vi "StartClone.vi"(7 "ShowPanel? (f)":bool, 8 "error in (no error)":errorcluster, 10 "ModuleName":string="unnamed", 11 "VI Refnum":refnum<vi>) -> (0 "error out":errorcluster, 1 "clBroadcastEvents":T1, 3 "ModuleAdmin":refnum<class "ModuleAdmin.lvclass">)   [LabVIEW 2018, in "SensorModule.lvlib"]
uses:
  SensorModule.lvlib
  SensorShared/clBroadcastEvents.ctl
  SensorShared/clEventType.ctl
  <userlib>/NIST/ModuleAdminLib/ModuleAdmin/ModuleAdmin.lvclass
  C:/Program Files (x86)/National Instruments/LabVIEW 2018/user.lib/NIST/ModuleAdminLib/ModuleAdminBase/ModuleAdminBase.lvclass
  <userlib>/NIST/ModuleAdminLib/ModuleAdmin/ModuleAdmin.lvclass/ModuleAdmin.ctl
  <userlib>/NIST/ModuleAdminLib/ModuleAdmin/Accessors/Write CloneRegRef.vi
  <userlib>/NIST/ModuleAdminLib/ModuleAdmin/Accessors/Write ShowPanel_.vi
  <vilib>/Utility/error.llb/Error Cluster From Error Code.vi
  <vilib>/ErrorRing/Error Ring.xnode
  SensorShared/SensorShared.lvlib
  <userlib>/NIST/ModuleAdminLib/ModuleAdminBase/ModuleAdminBase.lvclass
  <userlib>/NIST/ModuleAdminLib/CloneRegistration/CloneRegistration.lvclass
panel:
  # "If you want to add other Broadcast Events, open this typedef, copy an existing event and rename it to your event name.\n\nNext create an \"arg\" typedef for the  data and put it into PublicAPI/Arguments/Broadcasts\n\nAfter that, you will need to create a new roadcast vi in Protected/Broadcast.  Look at DidInit.vi or the reportError.vi as examples."
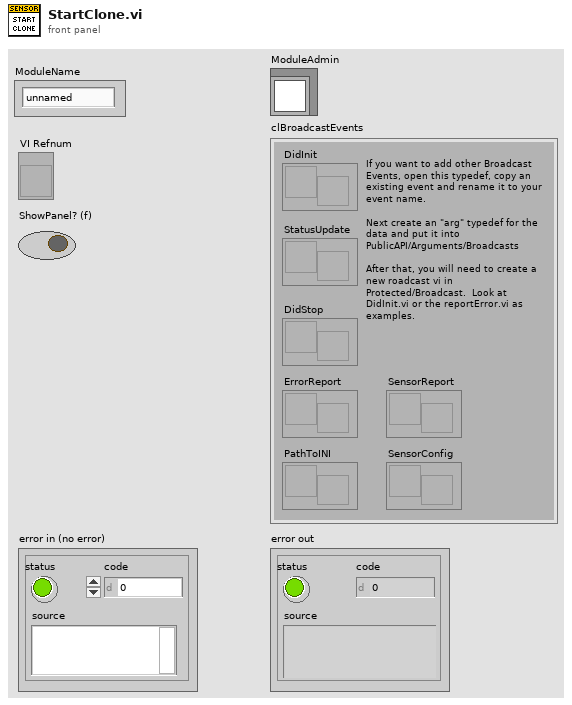
[diagram p1: front panel]
types:
  T1 = typedef "SensorShared.lvlib/clBroadcastEvents.ctl" = cluster{"DidInit":refnum<user-event>, "StatusUpdate":refnum<user-event>, "ErrorReport":refnum<user-event>, "DidStop":refnum<user-event>, "PathToINI":refnum<user-event>, "SensorReport":refnum<user-event>, "SensorConfig":refnum<user-event>}
  T2 = enum32{"Bad", "Idle", "Run top level", "Running"}
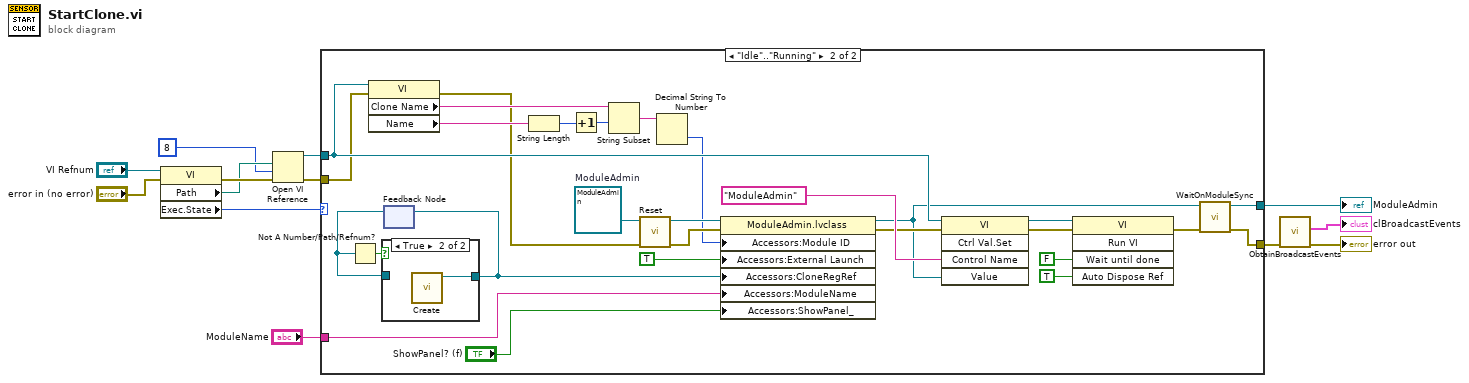
[diagram p0: block diagram]
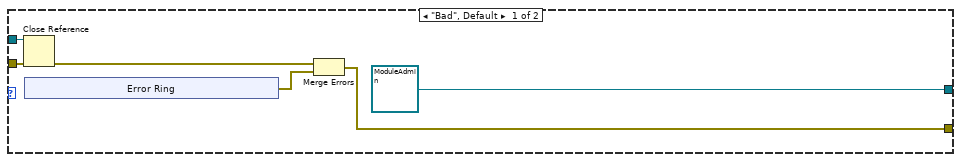
[diagram p2: hidden frame]
diagram:
  n1 = property class="VI"(reference="VI Refnum", error in="error in (no error)") -> (error out=w11:errorcluster, "Path"=w10:path, "Exec.State"=w12:T2)  [unwired: 1 out]
  n2 = Open VI Reference(vi path=w10, options=8, error in (no error)=w11) -> (vi reference=w8:refnum<vi>, error out=w9:errorcluster)  [unwired: 3 in]
  n3 = case shown="\"Idle\"..\"Running\"" w12 {
    tunnel: w9 -> [w19 w25]
    tunnel: w8 -> [w18 w42]
    tunnel: [w15 w32] -> w5
    tunnel: "ModuleName" -> [_ w31]
    tunnel: [refnum<class "ModuleAdmin.lvclass"> refnum ("ModuleAdmin") w30] -> w1
    frame "Bad", Default {
      n4 = Close Reference(reference=w18, error in (no error)=w19) -> (error out=w17:errorcluster)
      n5 = xnode "Error Ring"() -> ("error out"=w16:errorcluster)
      n6 = Merge Errors(w17, w16) -> (w15:errorcluster)
    }
    frame "Idle".."Running" {
      w46 = refnum<class "ModuleAdmin.lvclass"> refnum  # ModuleAdmin
      n7 = property class="VI"(reference=w42, error in=w25) -> (error out=w24:errorcluster, "Clone Name"=w48:string, "Name"=w51:string)  [unwired: 1 out]
      n8 = feedback #1() -> (w27:refnum<data-value>)  [unwired: 1 in]
      n9 = Not A Number/Path/Refnum?(number/path/refnum=w27) -> (NaN/Path/Refnum?=w28:bool)
      n10 = case shown="True" w28 {
        tunnel: [w52 w53] -> w26
        tunnel: w27 -> [w52 _]
        frame False {
        }
        frame True {
          n11 = call <userlib>:"Create.vi"() -> ("CloneRegRef"=w53:refnum<data-value>)  [unwired: 10 in, 1 out]
        }
      }
      n12 = feedback-in #1(w26) -> ()
      n13 = String Length(string=w51) -> (length=w50:i32)
      n14 = Increment(x=w50) -> (x+1=w49:i32)
      n15 = String Subset(string=w48, offset (0)=w49) -> (substring=w47:string)  [unwired: 1 in]
      n16 = call <userlib>:"Reset.vi"("error in (no error)"=w24, "Mod Admin in"=w46) -> ("error out"=w45:errorcluster, "Mod Admin out"=w44:refnum<class "ModuleAdmin.lvclass">)  [unwired: 8 in]
      n17 = Decimal String To Number(string=w47) -> (number=w34:i32)  [unwired: 2 in, 1 out]
      n18 = property class="ModuleAdmin.lvclass"(reference=w44, error in=w45, "Accessors:Module ID"=w34, "Accessors:External Launch"=TRUE ("External Launch"), "Accessors:CloneRegRef"=w26, "Accessors:ModuleName"=w31, "Accessors:ShowPanel_"="ShowPanel? (f)") -> (reference out=w33:refnum<class "ModuleAdmin.lvclass">, error out=w35:errorcluster)
      n19 = invoke class="VI" method="Ctrl Val.Set"(reference=w42, error in=w35, "Control Name"="ModuleAdmin", "Value"=w33) -> (reference out=w40:refnum<vi>, error out=w39:errorcluster)  [unwired: 1 in, 3 out]
      n20 = invoke class="VI" method="Run VI"(reference=w40, error in=w39, "Wait until done"=FALSE ("Wait Until Done"), "Auto Dispose Ref"=TRUE ("Auto Dispose Reference")) -> (error out=w36:errorcluster)  [unwired: 1 in, 4 out]
      n21 = call <userlib>:"WaitOnModuleSync.vi"("error in (no error)"=w36, "ModuleAdmin"=w33) -> ("error out"=w32:errorcluster, "ModuleAdmin"=w30:refnum<class "ModuleAdmin.lvclass">)  [unwired: 8 in]
    }
  }
  "ModuleAdmin" <- w1
  n22 = call "ObtainBroadcastEvents.vi"("error in (no error)"=w5) -> ("error out"=→"error out":errorcluster, "clBroadcastEvents"=→"clBroadcastEvents":T1)  [unwired: 9 in]
